vi "PhotonVision_Get_In_Range.vi"(6 "X Controller":dbl, 8 "Init":bool, 9 "AprilTagID":i32, 10 "Use AprilTag":bool, 11 "CameraName":string) -> (1 "Right Motor Value":dbl, 3 "Left Motor Value":dbl)   [LabVIEW 2019]
uses:
  <vilib>/Rock Robotics/WPI/ThirdParty/PhotonVisionLib/PhotonVisionLib.lvlib
  <vilib>/Rock Robotics/WPI/Joystick/WPI_JoystickArcadeMapping.vi
  <vilib>/Rock Robotics/WPI/ThirdParty/JAS_Junk/TrajLib/Trajectory_Library.lvlib
  <vilib>/Rock Robotics/Network Tables/NT Write Number.vi
  <vilib>/Rock Robotics/Network Tables/NT Write Boolean.vi
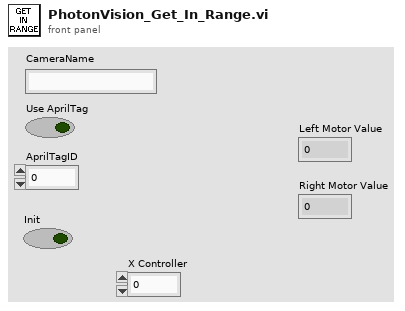
[diagram p1: front panel]
types:
  T1 = typedef "PhotonVisionLib.lvlib/PhotonPipelineResultType.ctl" = cluster{"Targets":T2[], "PhotonMultiTargetPNPResult":T8, "PhotonPipelineMetadata":T10}
  T2 = typedef "PhotonVisionLib.lvlib/PhotonTrackedTargetType.ctl" = cluster{"Yaw":dbl, "Pitch":dbl, "Area":dbl, "Skew":dbl, "MinAreaRectCorners":T3[], "BestCameraToTarget":T4, "FiducialId":i32, "AltCameraToTarget":T4, "PoseAmbiguity":dbl, "DetectedCorners":T3[], "ObjDetectId":i32, "ObjDetectConf":sgl}
  T3 = typedef "PhotonVisionLib.lvlib/TargetCornerType.ctl" = cluster{"X":dbl, "Y":dbl}
  T4 = typedef "Trajectory_Library.lvlib/TRANSFORM3D.ctl" = cluster{"TRANSLATION3D":T5, "ROTATION3D":T6, "XF":bool}
  T5 = typedef "Trajectory_Library.lvlib/TRANSLATION3D.ctl" = cluster{"X":dbl, "Y":dbl, "Z":dbl}
  T6 = typedef "Trajectory_Library.lvlib/ROTATION3D.ctl" = cluster{"Q_quaternion":T7}
  T7 = typedef "Trajectory_Library.lvlib/QUATERNION.ctl" = cluster{"R":dbl, "V":dbl[]}
  T8 = typedef "PhotonVisionLib.lvlib/PhotonMultiTargetPNPResultType.ctl" = cluster{"PhotonPNPResult":T9, "FiducialIDsUsed":i16[]}
  T9 = typedef "PhotonVisionLib.lvlib/PhotonPNPResultType.ctl" = cluster{"IsPresent":bool, "bestReprojErr":dbl, "altReprojErr":dbl, "ambiguity":dbl, "Best":T4, "Alt":T4}
  T10 = typedef "PhotonVisionLib.lvlib/PhotonPipelineMetadataType.ctl" = cluster{"CaptureTimestampMicros":i64, "PublishTimestampMicros":i64, "SequenceID":i64, "TimeSinceLastPong":i64}
  T11 = typedef "Trajectory_Library.lvlib/PID_ADV_LIMITS.ctl" = cluster{"MaxInput":dbl, "MinInput":dbl, "Continuous":bool, "MaxOutput":dbl, "MinOutput":dbl}
  T12 = typedef "Trajectory_Library.lvlib/PID_ADV_TUNING.ctl" = cluster{"Kf":dbl, "Kp":dbl, "Ki":dbl, "Kd":dbl, "MaximumIntegral":dbl, "MinimumIntegral":dbl, "Filter Derivative":bool, "IntegralZone":dbl}
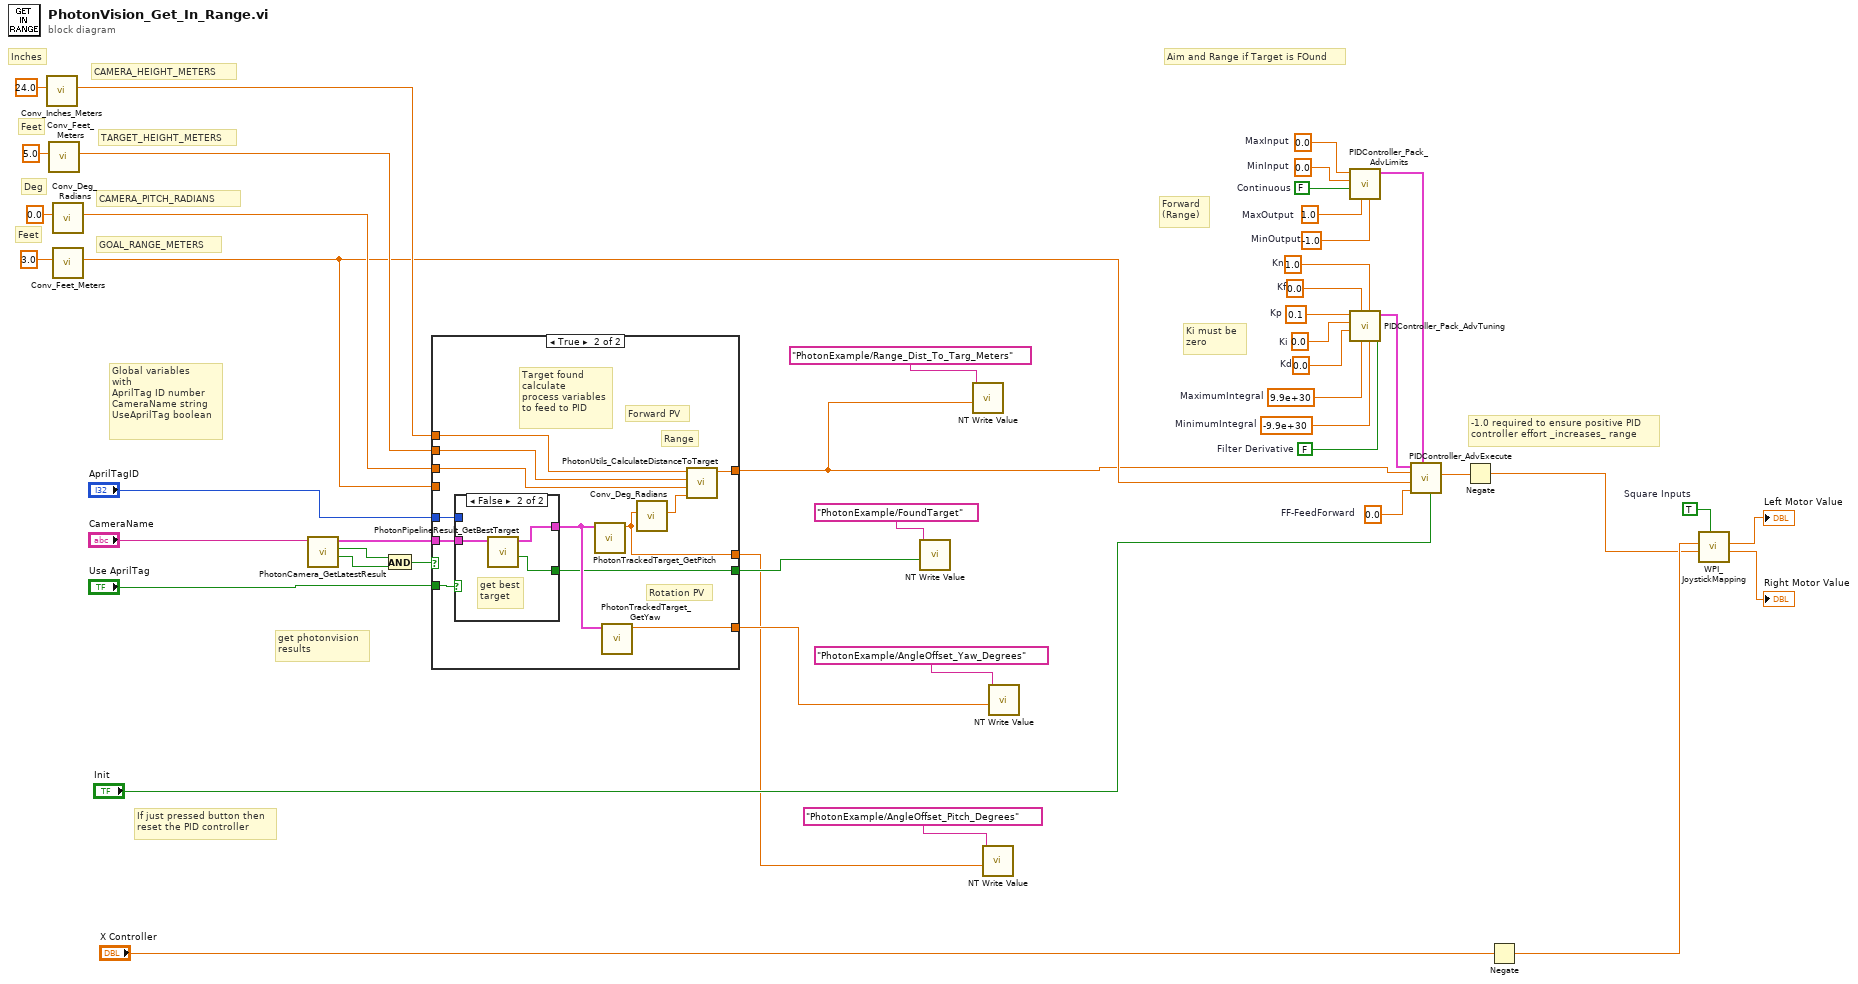
[diagram p0: block diagram]
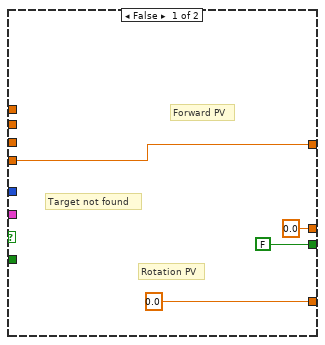
[diagram p2: hidden frame]
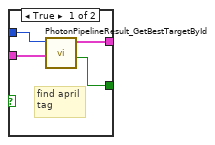
[diagram p3: hidden frame]
diagram:
  w34 = 0.0  # FF-FeedForward
  w17 = 1.0  # Kn
  w18 = 0.1  # Kp
  w19 = 0.0  # Ki
  w20 = 0.0  # Kd
  w21 = 0.0  # Kf
  w22 = 9.9e+30  # MaximumIntegral
  w23 = -9.9e+30  # MinimumIntegral
  w24 = FALSE  # Filter Derivative
  w26 = 0.0  # MinInput
  w27 = FALSE  # Continuous
  w28 = 1.0  # MaxOutput
  w25 = -1.0  # MinOutput
  w29 = 0.0  # MaxInput
  w14 = TRUE  # Square Inputs
  # "Global variables\nwith \nAprilTag ID number\nCameraName string\nUseAprilTag boolean"
  # "Feet"
  # "Deg"
  # "Feet"
  # "Inches"
  # "GOAL_RANGE_METERS"
  # "CAMERA_PITCH_RADIANS"
  # "TARGET_HEIGHT_METERS"
  # "CAMERA_HEIGHT_METERS"
  # "Aim and Range if Target is FOund"
  # "-1.0 required to ensure positive PID \ncontroller effort _increases_ range"
  # "Ki must be \nzero"
  # "If just pressed button then\nreset the PID controller"
  # "Forward \n(Range)"
  # "get photonvision\nresults"
  n1 = call <vilib>:"Conv_Inches_Meters.vi"("INCH"=24.0) -> ("Meters"=w47:dbl)  [unwired: 10 in]
  n2 = call <vilib>:"Conv_Feet_Meters.vi"("Feet"=5.0) -> ("Meters"=w46:dbl)  [unwired: 10 in]
  n3 = call <vilib>:"Conv_Deg_Radians.vi"("Degress"=0.0) -> ("Radians"=w45:dbl)  [unwired: 10 in]
  n4 = call <vilib>:"Conv_Feet_Meters.vi"("Feet"=3.0) -> ("Meters"=w44:dbl)  [unwired: 10 in]
  n5 = call <vilib>:"PhotonCamera_GetLatestResult.vi"("CameraName"="CameraName") -> ("New Data"=w3:bool, "HasTargets"=w4:bool, "PipelineResult"=w32:T1)  [unwired: 6 in, 2 out]
  n6 = And(x=w4, y=w3) -> (x .and. y?=w5:bool)
  n7 = case shown="True" w5 {
    tunnel: w32 -> [_ w63]
    tunnel: [w50 w60] -> w7
    tunnel: [0.0 w59] -> w9
    tunnel: w47 -> [_ w56]
    tunnel: w46 -> [_ w57]
    tunnel: w45 -> [_ w58]
    tunnel: w44 -> [w50 _]
    tunnel: "Use AprilTag" -> [_ w55]
    tunnel: [FALSE ("TargetFound") w54] -> w39
    tunnel: "AprilTagID" -> [_ w53]
    tunnel: [0.0 ("Pitch") w52] -> w1
    frame False {
      # "Forward PV"
      # "Rotation PV"
      # "Target not found"
    }
    frame True {
      # "Target found\ncalculate\nprocess variables\nto feed to PID"
      # "Range"
      # "Forward PV"
      # "Rotation PV"
      n8 = case shown="False" w55 {
        tunnel: w63 -> [w65 w70]
        tunnel: [w67 w69] -> w61
        tunnel: [w66 w68] -> w54
        tunnel: w53 -> [w64 _]
        frame True {
          # "find april\ntag"
          n9 = call <vilib>:"PhotonPipelineResult_GetBestTargetById.vi"("PhotonPipelineResult"=w65, "FiducialId"=w64) -> ("Target Found"=w66:bool, "PhotonTrackedTarget"=w67:T2)  [unwired: 7 in, 1 out]
        }
        frame False {
          # "get best\ntarget"
          n10 = call <vilib>:"PhotonPipelineResult_GetBestTarget.vi"("PhotonPipelineResult"=w70) -> ("TargetFound"=w68:bool, "PhotonTrackedTarget"=w69:T2)  [unwired: 9 in]
        }
      }
      n11 = call <vilib>:"PhotonTrackedTarget_GetPitch.vi"("TrackedTarget"=w61) -> ("Pitch"=w52:dbl)  [unwired: 10 in]
      n12 = call <vilib>:"PhotonTrackedTarget_GetYaw.vi"("TrackedTarget"=w61) -> ("Yaw"=w59:dbl)  [unwired: 10 in]
      n13 = call <vilib>:"Conv_Deg_Radians.vi"("Degress"=w52) -> ("Radians"=w62:dbl)  [unwired: 10 in]
      n14 = call <vilib>:"PhotonUtils_CalculateDistanceToTarget.vi"("TargetPitch_Radians"=w62, "CameraPitch_Radians"=w58, "TargetHeight_Meters"=w57, "CameraHeight_Meters"=w56) -> ("DistanceToTarget_Meters"=w60:dbl)  [unwired: 7 in]
    }
  }
  n15 = call-poly <vilib>:"NT Write Value.vi"("value"=w39, "name"="PhotonExample/FoundTarget" ("Name")) -> ()  [unwired: 9 in, 1 out]
  n16 = call-poly <vilib>:"NT Write Value.vi"("value"=w7, "name"="PhotonExample/Range_Dist_To_Targ_Meters" ("Name")) -> ()  [unwired: 9 in, 1 out]
  n17 = call-poly <vilib>:"NT Write Value.vi"("value"=w1, "name"="PhotonExample/AngleOffset_Pitch_Degrees" ("Name")) -> ()  [unwired: 9 in, 1 out]
  n18 = call-poly <vilib>:"NT Write Value.vi"("value"=w9, "name"="PhotonExample/AngleOffset_Yaw_Degrees" ("Name")) -> ()  [unwired: 9 in, 1 out]
  n19 = call <vilib>:"PIDController_Pack_AdvLimits.vi"("MinOutput"=w25, "MaxOutput"=w28, "Continuous"=w27, "MinInput"=w26, "MaxInput"=w29) -> ("Adv PID Limits"=w31:T11)  [unwired: 6 in]
  n20 = call <vilib>:"PIDController_Pack_AdvTuning.vi"("Filter Derivative"=w24, "MinimumIntegral"=w23, "Kn"=w17, "MaximumIntegral"=w22, "Kf"=w21, "Kd"=w20, "Ki"=w19, "Kp"=w18) -> ("Adv PID Tuning"=w30:T12)  [unwired: 3 in]
  n21 = call <vilib>:"PIDController_AdvExecute.vi"("Reset"="Init", "Adv PID Limits"=w31, "FF-FeedForward"=w34, "SP-SetPoint"=w44, "PV-Measurement"=w7, "Adv PID Tuning"=w30) -> ("CO-ControlOutput"=w35:dbl)  [unwired: 3 in, 2 out]
  n22 = Negate(x=w35) -> (-x=w36:dbl)
  n23 = Negate(x="X Controller") -> (-x=w37:dbl)
  n24 = call-poly <vilib>:"WPI_JoystickMapping.vi"("Square Inputs"=w14, "Y axis value"=w36, "X axis value"=w37) -> ("Right Motor Value"=→"Right Motor Value":dbl, "Left Motor Value"=→"Left Motor Value":dbl)  [unwired: 7 in]
